vi "Intan_parseDataStream_128ch.vi"(0 "1-D  data in":u16[](array[numeric]), 5 "bitMaskI16":i16[](array[numeric]), 7 "NumStreamCluster":T1, 9 "N data scans to read":i32=1) -> (3 "fragmented frame read":bool, 4 "2d ADCdata_array out_ampA_and_B":u16[][](array[numeric]), 6 "Vflex (V) out":dbl[](array[numeric]), 8 "Nscans read":i32, 10 "aux_cmd_array A":i16[][](array[numeric]), 11 "bytes parsed per scan":i32=148, 12 "ADXL analog data out":u16[][](array[numeric]), 13 "Vdd (V) out":dbl[](array[numeric]), 14 "Nscans underflow":bool, 15 "MagicNumOut":i32[](array[numeric]))   [LabVIEW 2020]
doc: "Reformats a 1d array of U16 Intan data (written by Teensy to serial port) into a 2-D array of data.\nThis takes Nscans worth of data, each with 36 words (= 72 bytes) worth of data, and reformats into 3 arrays:\n1. 'IN' = [73, 78] ascii values from auxiliary commands (this can be checked to verify data link)\n2. 32 bit timestamp (microseconds)\n3. Nchans (=32 for now) U16s for ADC data, with data formatted as Nchans x Nsamps\n\nRead error indicators suggest possible mis-read/mis-handling of data"
panel:
  out "Vflex binary":u16[](array[numeric])
  out "numElements":u16
  out "Vdd binary":u16[](array[numeric])
  out "timestamp_array":i32[](array[numeric])
  # "2-D data output"
  # "Data streaming format:\nFirst and last elements are always 'I' from amp A, and 22379 (magic num). Contents, in between depends on bit mask as follows;\n[0-31] amp A chans\n[32-63] amp B chans\n[64-95] amp C chans\n[96 - 127] amp D chans\n[128-130] accel (ax,ay,az)\n[131] Vbat (amp power supply)\n[132-159]: invalid (ignored)\n---------------------------------\nNote: Timestamps (4 bytes) and remaining intan aux_cmd bytes (8 bytes) are NOT transmitted in serial stream. This is done to save bandwidth for streaming more data.\n\n-JE 18 June 2019\nbitmask[0] and bitmask[142] should\nalways be set to stream per Teensy 3.6 firmware\n\n\n4 bytes aux_cmd_B\n4 bytes timestamp\n64 bytes ADC amp A\n64 bytes ADC amp B\n6 bytes ADXL (x,y,z)\n2 bytes sync bits (magic num)\n------------------\n148 bytes total"
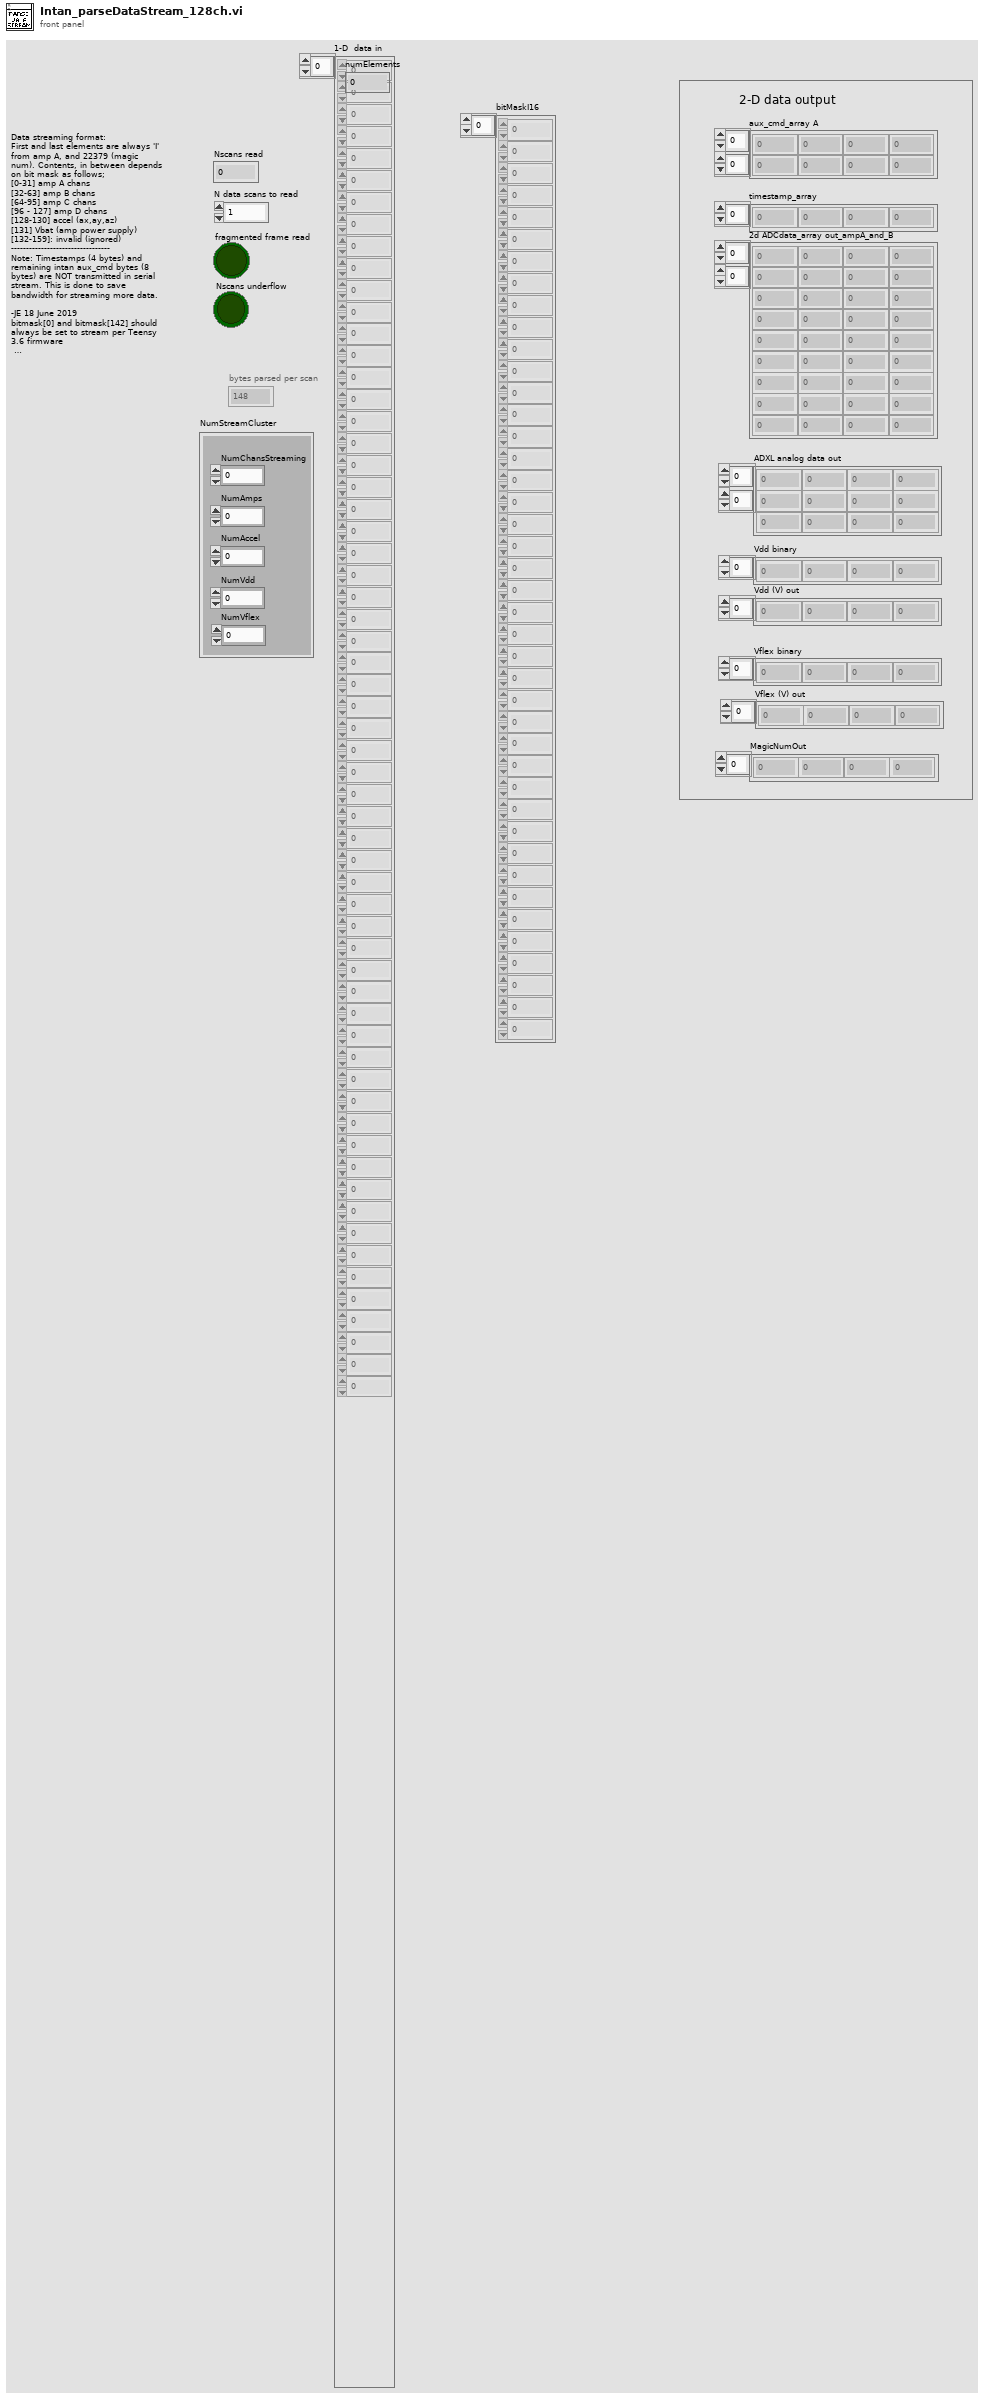
[diagram p1: front panel]
types:
  T1 = cluster{"NumChansStreaming":i16, "NumAmps":i32, "NumAccel":i32, "NumVdd":i32, "NumVflex":i32}
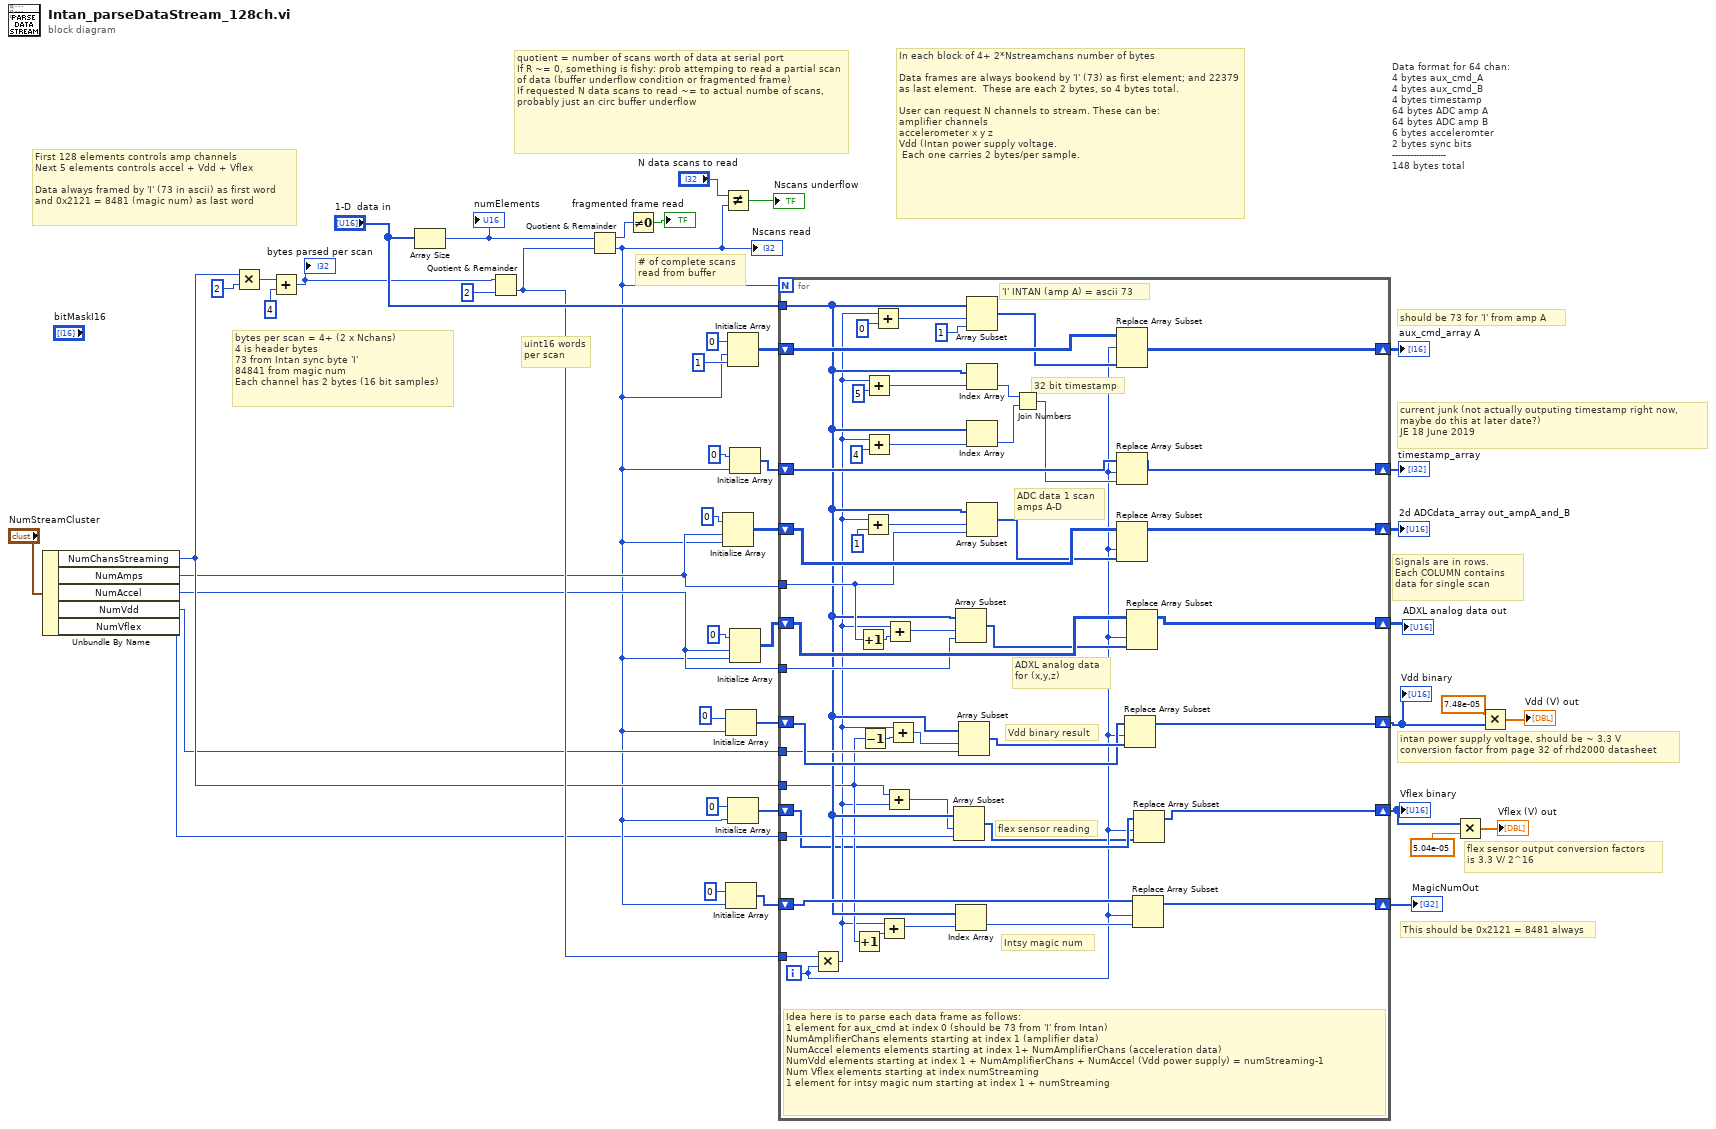
[diagram p0: block diagram]
diagram:
  # "flex sensor output conversion factors\nis 3.3 V/ 2^16"
  # "should be 73 for 'I' from amp A"
  # "current junk (not actually outputing timestamp right now,\nmaybe do this at later date?)\nJE 18 June 2019"
  # "intan power supply voltage, should be ~ 3.3 V\nconversion factor from page 32 of rhd2000 datasheet"
  # "bytes per scan = 4+ (2 x Nchans)\n4 is header bytes\n73 from Intan sync byte 'I'\n84841 from magic num\nEach channel has 2 bytes (16 bit samples)"
  # "First 128 elements controls amp channels\nNext 5 elements controls accel + Vdd + Vflex\n\nData always framed by 'I' (73 in ascii) as first word\nand 0x2121 = 8481 (magic num) as last word"
  # "This should be 0x2121 = 8481 always"
  # "Data format for 64 chan:\n4 bytes aux_cmd_A\n4 bytes aux_cmd_B\n4 bytes timestamp\n64 bytes ADC amp A\n64 bytes ADC amp B\n6 bytes acceleromter\n2 bytes sync bits\n------------------\n148 bytes total"
  # "# of complete scans\nread from buffer"
  # "Signals are in rows.\nEach COLUMN contains\ndata for single scan"
  # "In each block of 4+ 2*Nstreamchans number of bytes\n\nData frames are always bookend by 'I' (73) as first element; and 22379 as last element.  These are each 2 bytes, so 4 bytes total.\n\nUser can request N channels to stream. These can be:\namplifier channels\naccelerometer x y z\nVdd (Intan power supply voltage. \n Each one carries 2 bytes/per sample."
  # "quotient = number of scans worth of data at serial port \nIf R ~= 0, something is fishy: prob attemping to read a partial scan of data (buffer underflow condition or fragmented frame)\nIf requested N data scans to read ~= to actual numbe of scans, probably just an circ buffer underflow"
  # "uint16 words per scan"
  n1 = Unbundle By Name("NumStreamCluster") -> ("NumChansStreaming"=w11:i16, "NumAmps"=w10:i32, "NumAccel"=w9:i32, "NumVdd"=w8:i32, "NumVflex"=w4:i32)
  n2 = Multiply(x=w11, y=2) -> (x*y=w20:i32)
  n3 = Add(x=w20, y=4) -> (x+y=w18:i32)
  "bytes parsed per scan" <- w18
  n4 = Array Size(array="1-D  data in") -> (size(s)=w44:i32)
  "numElements" <- w44
  n5 = Quotient & Remainder(x=w18, y=2) -> (floor(x/y)=w40:i32)  [unwired: 1 out]
  n6 = Quotient & Remainder(x=w44, y=w40) -> (x-y*floor(x/y)=w43:i32, floor(x/y)=w6:i32)
  "Nscans read" <- w6
  n7 = Not Equal To 0?(x=w43) -> (x != 0?=→"fragmented frame read":bool)
  n8 = Not Equal?(x="N data scans to read", y=w6) -> (x != y?=→"Nscans underflow":bool)
  n9 = Initialize Array(u16 0 ("element"), w10, w6) -> (w33:u16[][])
  n10 = Initialize Array(u16 0 ("element"), w6) -> (w16:u16[])
  n11 = Initialize Array(0 ("element"), w6) -> (w24:i32[])
  n12 = Initialize Array(0 ("element"), w6, 1 ("dimension size")) -> (w35:i32[][])
  n13 = Initialize Array(u16 0 ("element"), w6) -> (w5:u16[])
  n14 = Initialize Array(0 ("element"), w6) -> (w34:i32[])
  n15 = Initialize Array(u16 0 ("element"), w9, w6) -> (w26:u16[][])
  n16 = for {
    N: w6 -> [_]
    tunnel: "1-D  data in" -> [w54]
    tunnel: w40 -> [w90]
    tunnel: w10 -> [w62]
    shift-right: [w77] -> w29
    shift-left: w34 -> [w80]
    shift-right: [w79] -> w30
    shift-left: w35 -> [w81]
    shift-right: [w76] -> w28
    shift-left: w33 -> [w78]
    shift-right: [w69] -> w25
    shift-left: w26 -> [w71]
    shift-right: [w68] -> w22
    shift-left: w24 -> [w67]
    tunnel: w9 -> [w64]
    tunnel: w11 -> [w51]
    shift-right: [w58] -> w15
    shift-left: w16 -> [w59]
    tunnel: w8 -> [w57]
    shift-right: [w49] -> w2
    shift-left: w5 -> [w48]
    tunnel: w4 -> [w53]
    i -> [w47]
    # "flex sensor reading"
    # "Intsy magic num"
    # "Idea here is to parse each data frame as follows:\n1 element for aux_cmd at index 0 (should be 73 from 'I' from Intan)\nNumAmplifierChans elements starting at index 1 (amplifier data)\nNumAccel elements elements starting at index 1+ NumAmplifierChans (acceleration data)\nNumVdd elements starting at index 1 + NumAmplifierChans + NumAccel (Vdd power supply) = numStreaming-1\nNum Vflex elements starting at index numStreaming \n1 element for intsy magic num starting at index 1 + numStreaming"
    # "Vdd binary result"
    # "ADXL analog data\nfor (x,y,z)"
    # "ADC data 1 scan\namps A-D"
    # "'I' INTAN (amp A) = ascii 73"
    # "32 bit timestamp"
    n17 = Multiply(x=w90, y=w47) -> (x*y=w50:i32)
    n18 = Increment(x=w51) -> (x+1=w61:i16)
    n19 = Increment(x=w62) -> (x+1=w63:i32)
    n20 = Decrement(x=w51) -> (x-1=w55:i16)
    n21 = Add(x=w50, y=1 ("index")) -> (x+y=w82:i32)
    n22 = Add(x=w50, y=5 ("index")) -> (x+y=w84:i32)
    n23 = Add(x=w50, y=4 ("index")) -> (x+y=w83:i32)
    n24 = Add(x=w50, y=0 ("index")) -> (x+y=w85:i32)
    n25 = Add(x=w50, y=w61) -> (x+y=w66:i32)
    n26 = Add(x=w51, y=w50) -> (x+y=w52:i32)
    n27 = Add(x=w50, y=w63) -> (x+y=w72:i32)
    n28 = Add(x=w50, y=w55) -> (x+y=w56:i32)
    n29 = Array Subset(array=w54, index=w52, length=w53) -> (w46:u16[])
    n30 = Array Subset(array=w54, index=w72, length=w64) -> (w70:u16[])
    n31 = Index Array(array=w54, index=w66) -> (element=w65:u16)
    n32 = Array Subset(array=w54, index=w56, length=w57) -> (w60:u16[])
    n33 = Array Subset(array=w54, index=w85, length=1) -> (w75:u16[])
    n34 = Index Array(array=w54, index=w84) -> (element=w92:u16)
    n35 = Index Array(array=w54, index=w83) -> (element=w91:u16)
    n36 = Array Subset(array=w54, index=w82, length=w62) -> (w73:u16[])
    n37 = Join Numbers(hi=w92, lo=w91) -> ((hi.lo)=w74:u32)
    n38 = Replace Array Subset(array=w81, new element=w75, index (row)=w47) -> (w79:i32[][])  [unwired: 1 in]
    n39 = Replace Array Subset(array=w80, new element=w74, index=w47) -> (w77:i32[])
    n40 = Replace Array Subset(array=w78, new element=w73, index (col)=w47) -> (w76:u16[][])  [unwired: 1 in]
    n41 = Replace Array Subset(array=w59, new element=w60, index=w47) -> (w58:u16[])
    n42 = Replace Array Subset(array=w71, new element=w70, index (col)=w47) -> (w69:u16[][])  [unwired: 1 in]
    n43 = Replace Array Subset(array=w67, new element=w65, index=w47) -> (w68:i32[])
    n44 = Replace Array Subset(array=w48, new element=w46, index=w47) -> (w49:u16[])
  }
  "aux_cmd_array A" <- w30
  "timestamp_array" <- w29
  "2d ADCdata_array out_ampA_and_B" <- w28
  "ADXL analog data out" <- w25
  "MagicNumOut" <- w22
  "Vdd binary" <- w15
  "Vflex binary" <- w2
  n45 = Multiply(x=w2, y=5.04e-05) -> (x*y=→"Vflex (V) out":dbl[])
  n46 = Multiply(x=7.48e-05 ("element"), y=w15) -> (x*y=→"Vdd (V) out":dbl[])
